vi "Shooter Tilter.vi"(11 "numericInput":i32) -> ()   [LabVIEW 2012]
panel:
  in  "motorSpeed":dbl
  in  "deadZone":dbl
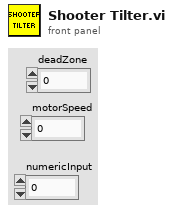
[diagram p1: front panel]
types:
  T1 = typedef "WPI_AnalogChannelDevRef.ctl" = cluster{"DevStatus":errorcluster, "Analog Module":T2, "Analog Channel":T3}
  T2 = typedef "FPGA_TypedefAnalogModule.ctl" = enum16{"Analog Module 1", "Analog Module 2"}
  T3 = typedef "FPGA_AIChannel.ctl" = enum8{"AI 1", "AI 2", "AI 3", "AI 4", "AI 5", "AI 6", "AI 7", "AI 8", "Invalid"}
  T4 = typedef "WPI_MotorControlDeviceRef.ctl" = cluster{"DeviceStatus":errorcluster, "Type":enum16{"PWM", "CAN"}, "PWM":cluster{"Digital Module":T5, "PWM Channel":T6, "DeadBand":T7}, "CAN":cluster{"Device Number":u8, "Control Mode":T8, "Semaphore":T9, "Max Vout":dbl}, "Invert":bool, "TransformRef":T10, "InvTransformRef":T10}
  T5 = typedef "FPGA_TypedefDigitalModule.ctl" = enum16{"Digital Module 1", "Digital Module 2"}
  T6 = typedef "FPGA_DIOPWMChannel.ctl" = enum8{"PWM 1", "PWM 2", "PWM 3", "PWM 4", "PWM 5", "PWM 6", "PWM 7", "PWM 8", "PWM 9", "PWM 10", "Invalid"}
  T7 = typedef "WPI_PWMDeadband.ctl" = cluster{"Name":string, "maxPositivePwm":i32, "minPositivePwm":i32, "centerPwm":i32, "maxNegativePwm":i32, "minNegativePwm":i32, "angularRange":u16}
  T8 = typedef "WPI_CANJaguar_ControlMode.ctl" = enum8{"Percent VBus", "Current", "Speed", "Position", "Voltage"}
  T9 = typedef "Semaphore RefNum" = refnum<k1>
  T10 = typedef "WPI_PWMTransform_ConPane.ctl" = refnum<vi>
  T11 = typedef "WPI_DigitalInputDevRef.ctl" = cluster{"DevStatus":errorcluster, "DIO Channel":T12, "Digital Module":T5}
  T12 = typedef "FPGA_DIOChannel.ctl" = enum8{"DIO 1", "DIO 2", "DIO 3", "DIO 4", "DIO 5", "DIO 6", "DIO 7", "DIO 8", "DIO 9", "DIO 10", "DIO 11", "DIO 12", "DIO 13", "DIO 14", "Invalid"}
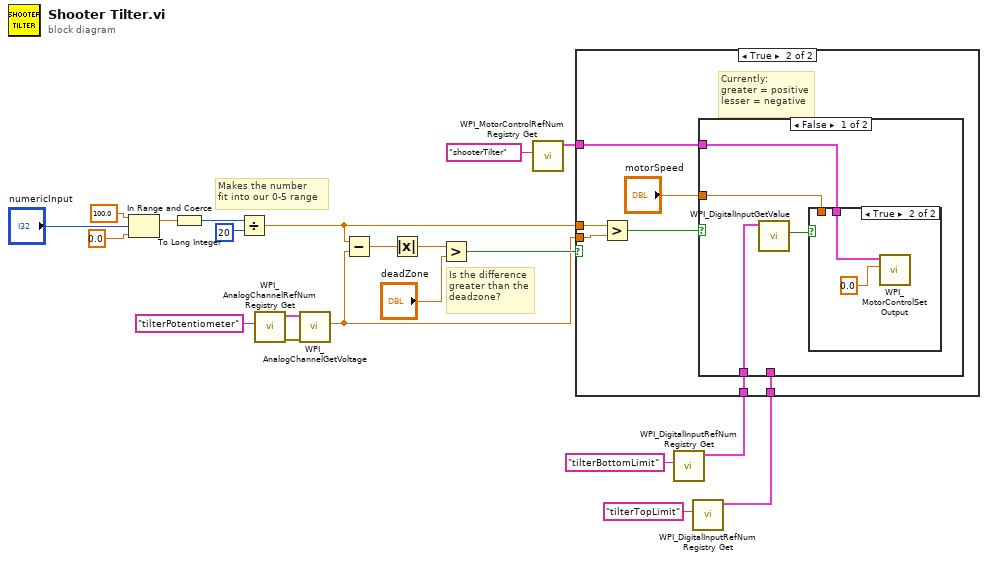
[diagram p0: block diagram]
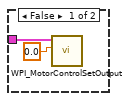
[diagram p2: hidden frame]
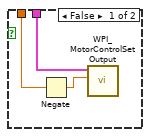
[diagram p3: hidden frame]
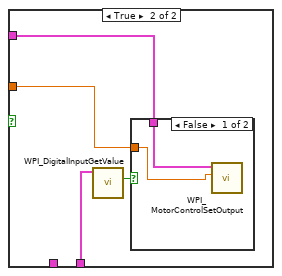
[diagram p4: hidden frame]
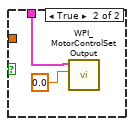
[diagram p5: hidden frame]
diagram:
  # "Makes the number\nfit into our 0-5 range"
  # "Is the difference\ngreater than the\ndeadzone?"
  n1 = In Range and Coerce(upper limit=100.0, x="numericInput", lower limit=0.0) -> (coerced(x)=w18:dbl)  [unwired: 1 out]
  n2 = To Long Integer(number=w18) -> (32bit integer=w17:i32)
  n3 = Divide(x=w17, y=20) -> (x/y=w5:dbl)
  n4 = call <vilib>:"WPI_AnalogChannelRefNum Registry Get.vi"("refnum name"="tilterPotentiometer") -> ("error out"=w14:errorcluster, "AIDeviceRef"=w13:T1)  [unwired: 9 in]
  n5 = call <vilib>:"WPI_AnalogChannelGetVoltage.vi"("error in (no error)"=w14, "AIDeviceRef"=w13) -> ("Voltage"=w7:dbl)  [unwired: 7 in, 2 out]
  n6 = Subtract(x=w5, y=w7) -> (x-y=w11:dbl)
  n7 = Absolute Value(x=w11) -> (abs(x)=w10:dbl)
  n8 = Greater?(x=w10, y="deadZone") -> (0:w9:bool)
  n9 = call <vilib>:"WPI_MotorControlRefNum Registry Get.vi"("refnum name"="shooterTilter") -> ("MotorControlDevRef"=w8:T4)  [unwired: 9 in, 1 out]
  n10 = call <vilib>:"WPI_DigitalInputRefNum Registry Get.vi"("refnum name"="tilterBottomLimit") -> ("DigitalInputDevRef"=w1:T11)  [unwired: 9 in, 1 out]
  n11 = call <vilib>:"WPI_DigitalInputRefNum Registry Get.vi"("refnum name"="tilterTopLimit") -> ("DigitalInputDevRef"=w2:T11)  [unwired: 9 in, 1 out]
  n12 = case shown="True" w9 {
    tunnel: w8 -> [w23 w29]
    tunnel: w7 -> [_ w30]
    tunnel: w5 -> [_ w27]
    tunnel: w2 -> [_ w26]
    tunnel: w1 -> [_ w25]
    frame False {
      n13 = call <vilib>:"WPI_MotorControlSetOutput.vi"("Output"=0.0, "MotorControlDevRef"=w23) -> ()  [unwired: 7 in, 3 out]
    }
    frame True {
      # "Currently:\ngreater = positive\nlesser = negative"
      n14 = Greater?(x=w27, y=w30) -> (0:w28:bool)
      n15 = case shown="False" w28 {
        tunnel: w29 -> [w32 w41]
        tunnel: w26 -> [_ w43]
        tunnel: w25 -> [w34 _]
        tunnel: "motorSpeed" -> [w31 w40]
        frame False {
          n16 = call <vilib>:"WPI_DigitalInputGetValue.vi"("DigitalInputDevRef"=w34) -> ("Value"=w33:bool)  [unwired: 8 in, 2 out]
          n17 = case shown="True" w33 {
            tunnel: w32 -> [w37 w39]
            tunnel: w31 -> [w36 _]
            frame False {
              n18 = Negate(x=w36) -> (-x=w35:dbl)
              n19 = call <vilib>:"WPI_MotorControlSetOutput.vi"("Output"=w35, "MotorControlDevRef"=w37) -> ()  [unwired: 7 in, 3 out]
            }
            frame True {
              n20 = call <vilib>:"WPI_MotorControlSetOutput.vi"("Output"=0.0, "MotorControlDevRef"=w39) -> ()  [unwired: 7 in, 3 out]
            }
          }
        }
        frame True {
          n21 = call <vilib>:"WPI_DigitalInputGetValue.vi"("DigitalInputDevRef"=w43) -> ("Value"=w42:bool)  [unwired: 8 in, 2 out]
          n22 = case shown="False" w42 {
            tunnel: w41 -> [w45 w47]
            tunnel: w40 -> [w44 _]
            frame False {
              n23 = call <vilib>:"WPI_MotorControlSetOutput.vi"("Output"=w44, "MotorControlDevRef"=w45) -> ()  [unwired: 7 in, 3 out]
            }
            frame True {
              n24 = call <vilib>:"WPI_MotorControlSetOutput.vi"("Output"=0.0, "MotorControlDevRef"=w47) -> ()  [unwired: 7 in, 3 out]
            }
          }
        }
      }
    }
  }
